vi "Start Executions.vi"(8 "error in (no error)":errorcluster, 10 "Main Continer":refnum<vi>, 11 "Application in":refnum<data-value>) -> (0 "error out":errorcluster, 3 "Application out":refnum<data-value>)   [LabVIEW 2015, in "Application.lvclass"]
uses:
  Application.lvclass
  Plugin.lvclass
  Project.lvclass
  Execution.lvclass
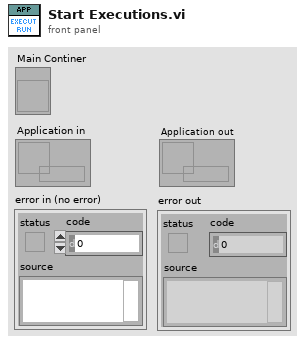
[diagram p1: front panel]
types:
  T1 = cluster{"Order":enum16{"LeftRight", "TopDown"}, "Row":i32, "Column":i32, "Margin":i32}
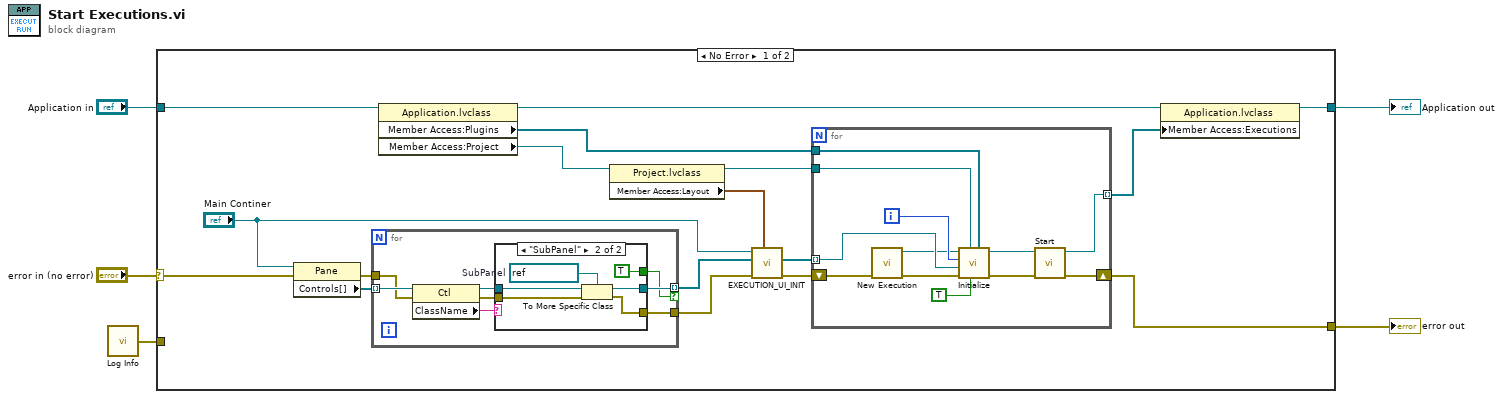
[diagram p0: block diagram]
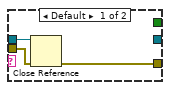
[diagram p2: hidden frame]
diagram:
  n1 = call "Log Info.vi"() -> ("error out"=w3:errorcluster)  [unwired: 5 in]
  n2 = case shown="No Error" "error in (no error)" {
    selector: "error in (no error)" -> [w11 w53]
    tunnel: [w20 w53] -> w4
    tunnel: [w21 w52] -> w1
    tunnel: "Application in" -> [w9 w52]
    tunnel: w3 -> [_ _]
    frame No Error {
      n3 = property class="Pane"(reference="Main Continer", error in=w11) -> (error out=w15:errorcluster, "Controls[]"=w14:refnum<vi>[])  [unwired: 1 out]
      n4 = for {
        tunnel: w14 -> [w30] mode=indexing
        tunnel: w15 -> [w27]
        tunnel: [w25] -> w12 mode=indexing if=w24
        tunnel: [w23] -> w10
        n5 = property class="Ctl"(reference=w30, error in=w27) -> (reference out=w28:refnum<vi>, error out=w26:errorcluster, "ClassName"=w29:string)
        n6 = case shown="\"SubPanel\"" w29 {
          tunnel: w28 -> [w33 w38]
          tunnel: [_ w34] -> w25
          tunnel: [w32 w36] -> w23
          tunnel: [_ TRUE] -> w24
          tunnel: w26 -> [w31 w37]
          frame Default {
            n7 = Close Reference(reference=w33, error in (no error)=w31) -> (error out=w32:errorcluster)
          }
          frame "SubPanel" {
            w35 = refnum<vi> refnum  # SubPanel
            n8 = To More Specific Class(target class=w35, reference=w38, error in=w37) -> (specific class reference=w34:refnum<vi>, error out=w36:errorcluster)
          }
        }
      }
      n9 = property class="Application.lvclass"(reference=w9) -> (reference out=w6:refnum<data-value>, "Member Access:Plugins"=w7:refnum<class "Plugin.lvclass">[], "Member Access:Project"=w8:refnum<class "Project.lvclass">)  [unwired: 1 in, 1 out]
      n10 = property class="Project.lvclass"(reference=w8) -> (reference out=w16:refnum<class "Project.lvclass">, "Member Access:Layout"=w17:T1)  [unwired: 1 in, 1 out]
      n11 = call "EXECUTION_UI_INIT.vi"("Layout"=w17, "error in (no error)"=w10, "Execution Panels"=w12, "Container Panel"="Main Continer") -> ("error out"=w19:errorcluster, "Execution Panels In Use"=w22:refnum<vi>[])  [unwired: 6 in]
      n12 = for {
        tunnel: w22 -> [w51] mode=indexing
        shift-right: [w49] -> w20
        shift-left: w19 -> [w42]
        tunnel: [w48] -> w18 mode=indexing
        tunnel: w16 -> [w46]
        tunnel: w7 -> [w45]
        i -> [w50]
        n13 = call "New Execution.vi"("error in (no error)"=w42) -> ("error out"=w41:errorcluster, "Execution"=w40:refnum<data-value>)  [unwired: 9 in]
        n14 = call "Initialize.vi"("Plugins"=w45, "Enable"=TRUE, "Project"=w46, "error in (no error)"=w41, "Container"=w51, "Index"=w50, "Execution in"=w40) -> ("error out"=w43:errorcluster, "Execution out"=w44:refnum<data-value>)  [unwired: 3 in]
        n15 = call "Start.vi"("error in (no error)"=w43, "Execution in"=w44) -> ("error out"=w49:errorcluster, "Execution out"=w48:refnum<data-value>)  [unwired: 8 in]
      }
      n16 = property class="Application.lvclass"(reference=w6, "Member Access:Executions"=w18) -> (reference out=w21:refnum<data-value>)  [unwired: 1 in, 1 out]
    }
    frame Error {
    }
  }
  "error out" <- w4
  "Application out" <- w1
